vi "Regular Search and Replace All Fitable Contents In String.vi"(8 "error in (no error)":errorcluster, 9 "replace string (\"\")":string, 10 "regular expression (\"\")":string, 11 "Source(\"\")":string) -> (0 "error out":errorcluster, 3 "Changed Content(\"\")":string)   [LabVIEW 2015]
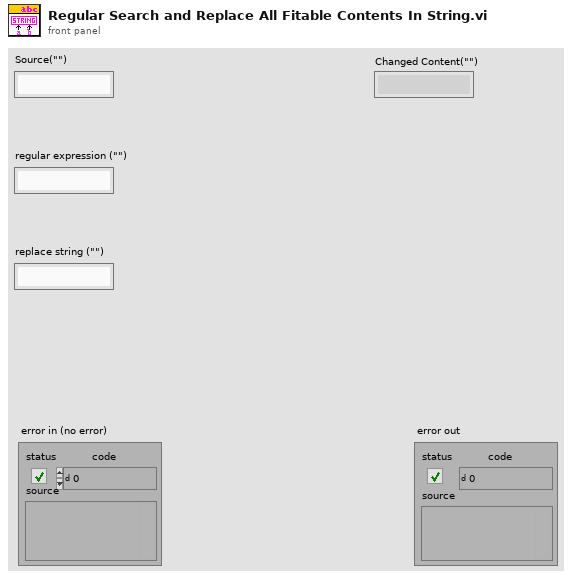
[diagram p1: front panel]
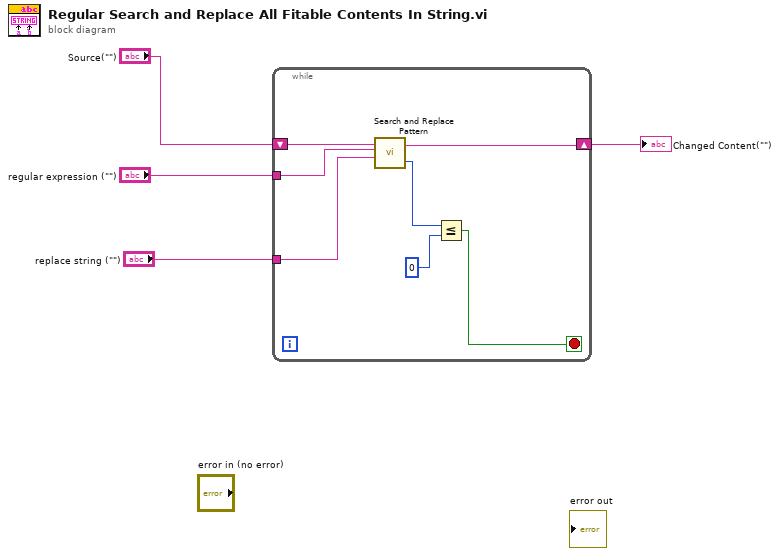
[diagram p0: block diagram]
diagram:
  n1 = while {
    shift-right: [w8] -> w1
    shift-left: "Source(\"\")" -> [w11]
    tunnel: "regular expression (\"\")" -> [w10]
    tunnel: "replace string (\"\")" -> [w9]
    stop <- w5 stop-if-true
    n2 = call <vilib>:"Search and Replace Pattern.vi"("string"=w11, "regular expression (\"\")"=w10, "replace string (\"\")"=w9) -> ("result string"=w8:string, "offset past match"=w7:i32)  [unwired: 2 in]
    n3 = Less Or Equal?(x=w7, y=0) -> (x <= y?=w5:bool)
  }
  "Changed Content(\"\")" <- w1
